vi "SignalMeasurementsFromFile.vi"() -> ()   [LabVIEW 2025]
panel:
  out "signal":waveform(dbl)(graph)
  out "error out":errorcluster
  out "max frequency":dbl
  out "signal power":dbl
  out "f0":dbl
  out "df":dbl
  out "magnitude":dbl[](graph)
  in  "error in":errorcluster
  in  "file path in":path
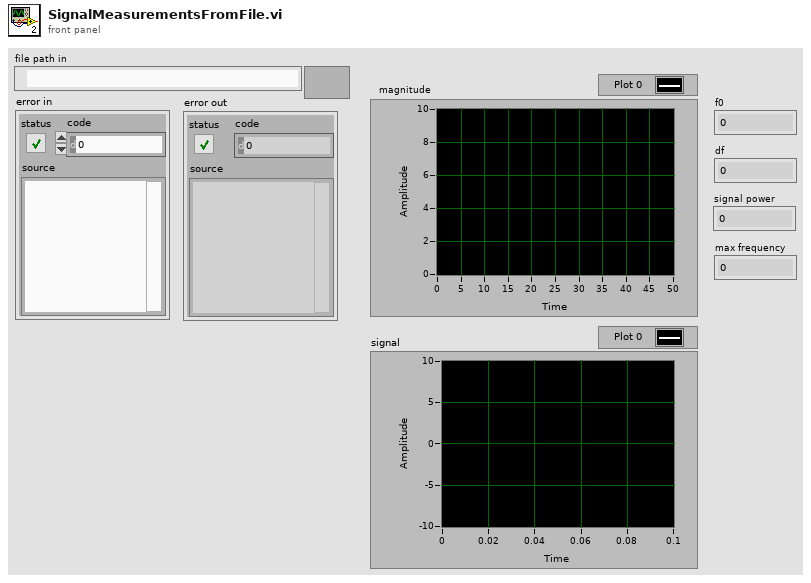
[diagram p1: front panel]
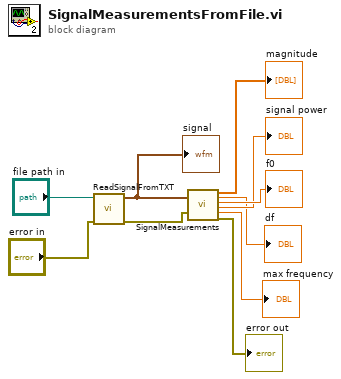
[diagram p0: block diagram]
diagram:
  n1 = call "ReadSignalFromTXT.vi"("error in"="error in", "file path in"="file path in") -> ("error out"=w10:errorcluster, "signal out"=w1:waveform(dbl))  [unwired: 8 in]
  "signal" <- w1
  n2 = call "SignalMeasurements.vi"("Waveform"=w1, "error in"=w10) -> ("magnitude"=→"magnitude":dbl[], "df"=→"df":dbl, "f0"=→"f0":dbl, "signal power"=→"signal power":dbl, "max frequency"=→"max frequency":dbl, "error out"=→"error out":errorcluster)  [unwired: 12 in]
